vi "EmptyH5ErrorStack.vi"() -> (0 "Empty Error Stack":T1[](array[typedef]))   [LabVIEW 2017]
uses:
  <vilib>/UPVI/lvhdf5/common.llb/HDF5 Error Cluster.ctl
panel:
  in  "HDF5 Error Cluster":T1
  # "LVHDF5 Toolkit\nCopyright (c) 2005-2013 by Jason D. Sommerville\nCopyright (c) 2014 by UPVI, LLC.\n\nThis use and distribution of this file is governed by the terms found in \nLICENSE.txt distributed with this toolkit and installed at\n <user.lib>\\_lvhdf5\\LICENSE.txt"
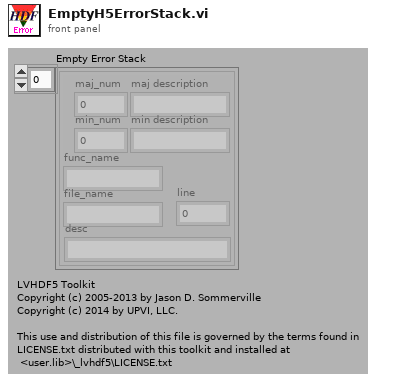
[diagram p1: front panel]
types:
  T1 = typedef "HDF5 Error Cluster.ctl" = cluster{"maj_num":i32, "min_num":i32, "func_name":string, "file_name":string, "line":u32, "desc":string, "maj description":string, "min description":string}
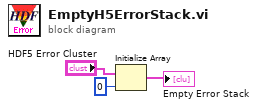
[diagram p0: block diagram]
diagram:
  n1 = Initialize Array("HDF5 Error Cluster", 0 ("dimension size")) -> (→"Empty Error Stack":T1[])
